vi "wcLED_topLvl.vi"(5 "which manipulator":T1(ring), 8 "error in (no error)":errorcluster, 10 "wc LED":bool, 11 "Pressure box control in":T2) -> (0 "error out":errorcluster, 3 "Pressure box control out":T2)   [LabVIEW 2015]
uses:
  controls/proportionAir_cmds.ctl
  controls/pressure_box_type.ctl
  controls/pressure_box_control.ctl
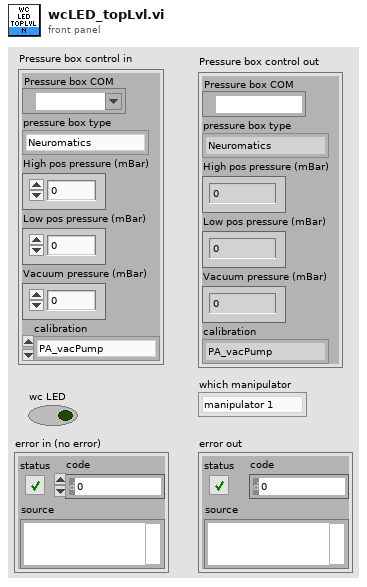
[diagram p1: front panel]
types:
  T1 = enum16{"manipulator 1", "manipulator 2", "manipulator 3", "manipulator 4"}
  T2 = typedef "pressure_box_control.ctl" = cluster{"Pressure box COM":refnum<visa-resource-name>, "pressure box type":T3, "High pos pressure (mBar)":dbl, "Low pos pressure (mBar)":dbl, "Vacuum pressure (mBar)":dbl, "calibration":enum16{"PA_vacPump", "PA_venturi", "Neuromatics", "ilyaRig", "mightenRig"}}
  T3 = typedef "pressure_box_type.ctl" = enum16{"Neuromatics", "ProportionAir", "Demo box", "N-ProportionAir"}
  T4 = typedef "proportionAir_cmds.ctl" = enum16{"Set P", "Switch to Atm", "Switch to Regulator", "Pulse", "WC"}
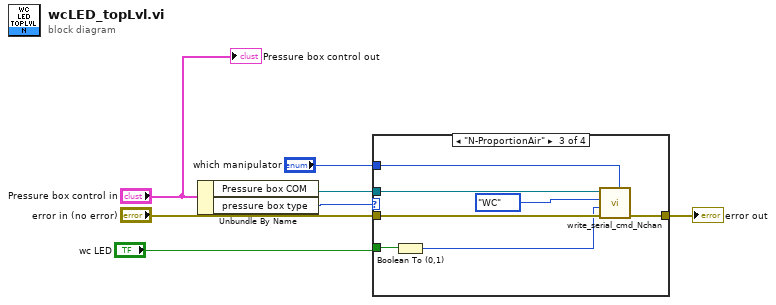
[diagram p0: block diagram]
diagram:
  n1 = Unbundle By Name("Pressure box control in") -> ("Pressure box COM"=w5:refnum<visa-resource-name>, "pressure box type"=w6:T3)
  n2 = case shown="\"N-ProportionAir\"" w6 {
    tunnel: "error in (no error)" -> [w8 w9 w16 w17]
    tunnel: [w8 w9 w15 w17] -> w4
    tunnel: w5 -> [_ _ w14 _]
    tunnel: "wc LED" -> [_ _ w11 _]
    tunnel: "which manipulator" -> [_ _ w13 _]
    frame "Neuromatics", Default {
    }
    frame "ProportionAir" {
    }
    frame "N-ProportionAir" {
      n3 = Boolean To (0,1)(Boolean=w11) -> (0, 1=w10:i16)
      n4 = call "write_serial_cmd_Nchan.vi"("which manipulator"=w13, "error in"=w16, "arg 1"=w10, "pressure command"=proportionAir_cmds."WC", "Pressure Box COM"=w14) -> ("error out"=w15:errorcluster)  [unwired: 5 in, 1 out]
    }
    frame "Demo box" {
    }
  }
  "error out" <- w4
  "Pressure box control out" <- "Pressure box control in"
